vi "Read config running.vi"(8 "error in (no error)":errorcluster, 11 "Acquisition in":refnum<class "Acquisition.lvclass">) -> (0 "error out":errorcluster, 2 "config running":bool, 3 "Acquisition out":refnum<class "Acquisition.lvclass">)   [LabVIEW 2018, in "Acquisition.lvclass"]
uses:
  Acquisition.lvclass
  Acquisition.lvclass/Acquisition.ctl
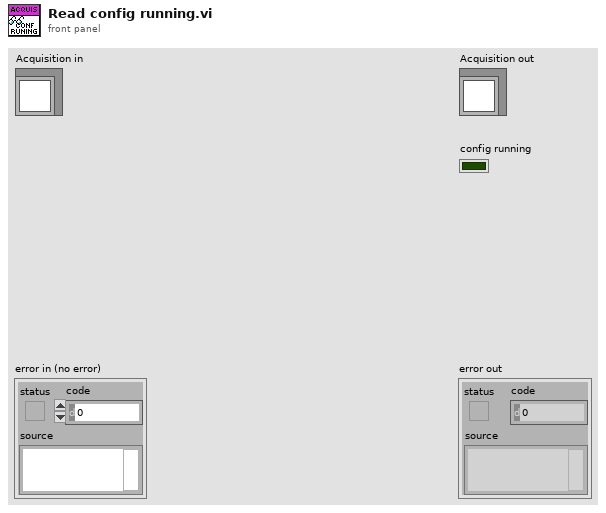
[diagram p1: front panel]
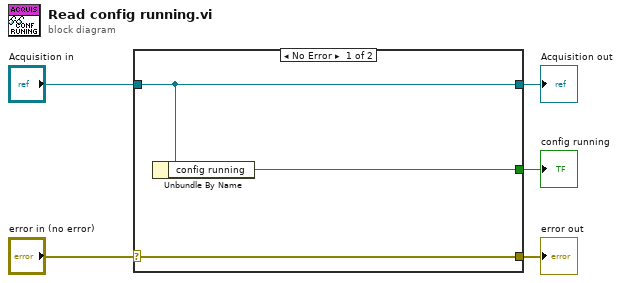
[diagram p0: block diagram]
diagram:
  n1 = case shown="No Error" "error in (no error)" {
    selector: "error in (no error)" -> [w8 w9]
    tunnel: [w8 w9] -> w4
    tunnel: [w7 w10] -> w2
    tunnel: "Acquisition in" -> [w7 w10]
    tunnel: [w6 _] -> w1
    frame No Error {
      n2 = Unbundle By Name(w7) -> ("config running"=w6:bool)
    }
    frame Error {
    }
  }
  "error out" <- w4
  "Acquisition out" <- w2
  "config running" <- w1
